vi "Defer Front Panel Updates.vi"(8 "error in (no error)":errorcluster, 10 "Defer":bool, 11 "Hex Viewer in":refnum<class "Hex Viewer.lvclass">) -> (0 "error out":errorcluster)   [LabVIEW 2021, in "Hex Viewer.lvclass"]
uses:
  Hex Viewer.lvclass
  Hex Viewer.lvclass/Hex Viewer.ctl
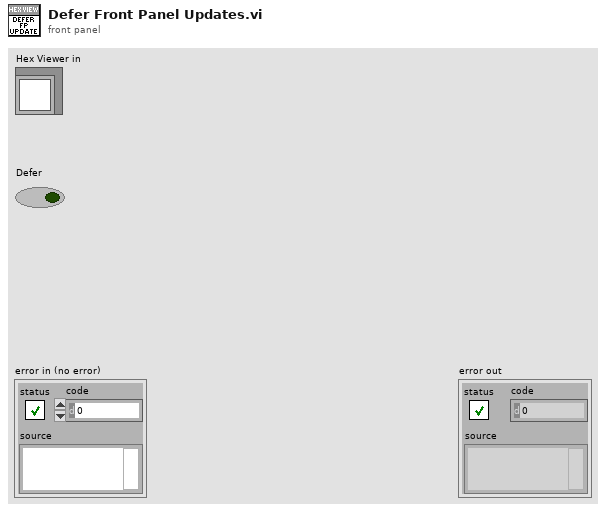
[diagram p1: front panel]
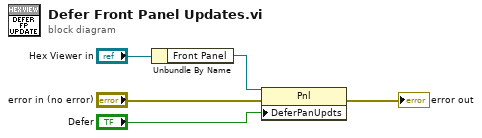
[diagram p0: block diagram]
diagram:
  n1 = Unbundle By Name("Hex Viewer in") -> ("Front Panel"=w2:refnum<vi>)
  n2 = property class="Pnl"(reference=w2, error in="error in (no error)", "DeferPanUpdts"="Defer") -> (error out=→"error out":errorcluster)  [unwired: 1 out]
